vi "GetChartArea.vi"(3 "Draw Area Size":T1) -> (0 "Chart Area Size":cluster{"Width":dbl, "Height":dbl}, 1 "Height":dbl)   [LabVIEW 2019, in "Zen Analytics.lvlib" / "Zen Analytics.lvclass"]
uses:
  Zen Analytics.lvclass
  <vilib>/Utility/miscctls.llb/LVBoundsTypeDef.ctl
types:
  T1 = typedef "LVBoundsTypeDef.ctl" = cluster{"Width":u32, "Height":u32}
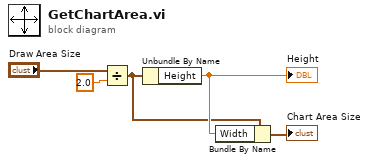
[diagram p0: block diagram]
diagram:
  n1 = Divide(x="Draw Area Size", y=2.0) -> (x/y=w3:cluster{"Width":dbl, "Height":dbl})
  n2 = Unbundle By Name(w3) -> ("Height"=w4:dbl)
  "Height" <- w4
  n3 = Bundle By Name(cluster=w3, "Width"=w4) -> (→"Chart Area Size":cluster{"Width":dbl, "Height":dbl})
